vi "Min Max Array.vi"(9 "Min Values":dbl[](array[numeric]), 10 "Input Array":dbl[](array[numeric]), 11 "Max Values":dbl[](array[numeric])) -> (1 "Min Values Out":dbl[](array[numeric]), 3 "Max Values Out":dbl[](array[numeric]))   [LabVIEW 2013, in "Super Simple Neural Network.lvlib"]
uses:
  Super Simple Neural Network.lvlib
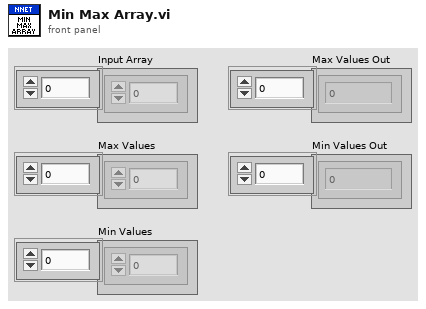
[diagram p1: front panel]
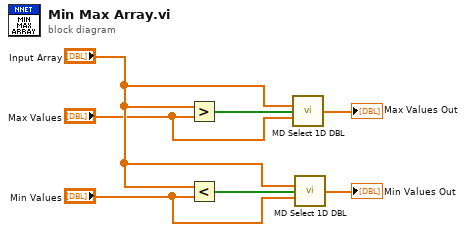
[diagram p0: block diagram]
diagram:
  n1 = Greater?(x="Input Array", y="Max Values") -> (0:w2:bool[])
  n2 = Less?(x="Input Array", y="Min Values") -> (x < y?=w4:bool[])
  n3 = call "MD Select 1D DBL.vi"("First Array"="Input Array", "Condition"=w2, "Second Array"="Max Values") -> ("Resulting Array"=→"Max Values Out":dbl[])  [unwired: 12 in]
  n4 = call "MD Select 1D DBL.vi"("First Array"="Input Array", "Condition"=w4, "Second Array"="Min Values") -> ("Resulting Array"=→"Min Values Out":dbl[])  [unwired: 12 in]
